vi "sim_MmW_GetAttributes.vi"(8 "error in (no error)":errorcluster, 10 "return data? (T)":bool=TRUE, 11 "reference in":refnum<class "sim_MmW.lvclass">) -> (0 "error out":errorcluster, 1 "attributes":T1={"RF config"={"TX.Frequency"=0.0, "TX.Gain"=-10.0, "TX.mmWave adapter"="mmWave1/0", "RX.Frequency"=76000000000.0, "RX.Gain"=0.0, "RX.mmWave adapter"="mmWave0/0"}, "RX samples"=0, "Downloaded Bursts"={}, "TX Fs"=0.0, "RX Fs"=0.0, "burst sequence"=[], "Burst mode"=enum."burst"} {"RF config"."RX.Frequency" format="%#_6pHz"; "RF config"."RX.Gain" format="%#_6fdb"; "RF config"."TX.Frequency" format="%#_6pHz"; "RF config"."TX.Gain" format="%#_6pHz"}, 2 "attributes ref":T4, 3 "reference out":refnum<class "sim_MmW.lvclass">)   [LabVIEW 2019, in "sim_MmW.lvclass"]
doc: "Returns a reference and if wanted the actual data values of the attributes. This method is used by the subclasses to access parent attributes."
uses:
  sim_MmW.lvclass
  C:/Program Files/National Instruments/LabVIEW 2019/vi.lib/addons/_AddQ/G#Object/G#Object.lvclass
  ObjectAttributesRef.ctl
  protected/ObjectAttributes.ctl
  mmWave HW Control/HW TXRX RF config cluster.ctl
  mmWave data_class/mmWave data.lvclass
  mmWave instrument_class/BurstMode.ctl
  sim_MmW.lvclass/sim_MmW.ctl
  <vilib>/addons/_AddQ/G#Object/G#Object.lvclass
  mmWave HW Control/mmWave HW Control.lvlib
  mmWave instrument_class/mmWave instrument.lvclass
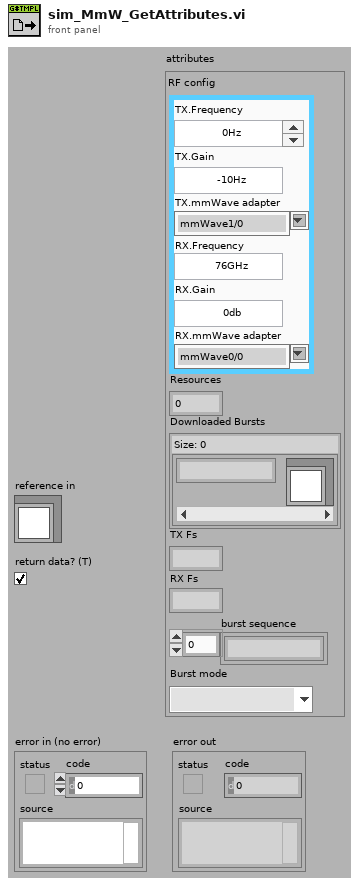
[diagram p1: front panel]
types:
  T1 = typedef "sim_MmW.lvclass/ObjectAttributes.ctl" = cluster{"RF config":T2, "RX samples":i32, "Downloaded Bursts":map{string, refnum<class "mmWave data.lvclass">}, "TX Fs":dbl, "RX Fs":dbl, "burst sequence":string[], "Burst mode":T3}
  T2 = typedef "mmWave HW Control.lvlib/HW TXRX RF config cluster.ctl" = cluster{"TX.Frequency":dbl, "TX.Gain":dbl, "TX.mmWave adapter":string, "RX.Frequency":dbl, "RX.Gain":dbl, "RX.mmWave adapter":string}
  T3 = typedef "mmWave instrument.lvclass/BurstMode.ctl" = enum16{"burst", "continuous"}
  T4 = typedef "sim_MmW.lvclass/ObjectAttributesRef.ctl" = refnum<data-value>
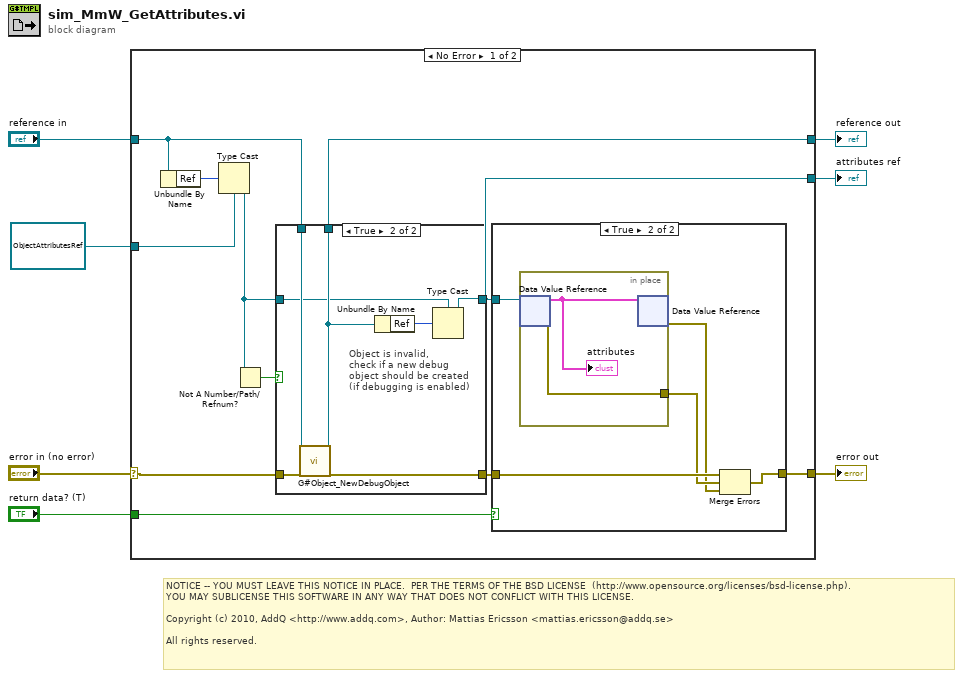
[diagram p0: block diagram]
diagram:
  # "NOTICE -- YOU MUST LEAVE THIS NOTICE IN PLACE.  PER THE TERMS OF THE BSD LICENSE  (http://www.opensource.org/licenses/bsd-license.php).\nYOU MAY SUBLICENSE THIS SOFTWARE IN ANY WAY THAT DOES NOT CONFLICT WITH THIS LICENSE.\n\nCopyright (c) 2010, AddQ <http://www.addq.com>, Author: Mattias Ericsson <mattias.ericsson@addq.se>\n\nAll rights reserved."
  n1 = case shown="No Error" "error in (no error)" {
    selector: "error in (no error)" -> [w14 w39]
    tunnel: [w17 w39] -> w6
    tunnel: [w11 w38] -> w4
    tunnel: "reference in" -> [w12 w38]
    tunnel: [w8 w37] -> w3
    tunnel: "return data? (T)" -> [w18 _]
    tunnel: T4 refnum ("attributes ref") -> [w10 w37]
    frame No Error {
      n2 = Unbundle By Name(w12) -> ("Ref"=w16:u32)
      n3 = Type Cast(type=w10, x=w16) -> (*(type *) &x=w9:T4)
      n4 = Not A Number/Path/Refnum?(number/path/refnum=w9) -> (NaN/Path/Refnum?=w13:bool)
      n5 = case shown="True" w13 {
        tunnel: [w21 w28] -> w15
        tunnel: w14 -> [w21 w27]
        tunnel: w12 -> [w20 w26]
        tunnel: [w20 w24] -> w11
        tunnel: w9 -> [w19 w23]
        tunnel: [w19 w22] -> w8
        frame False {
        }
        frame True {
          # "Object is invalid,\ncheck if a new debug\nobject should be created\n(if debugging is enabled)"
          n6 = call <vilib>:"G#Object_NewDebugObject.vi"("reference in"=w26, "error in (no error)"=w27) -> ("reference out"=w24:refnum<class "sim_MmW.lvclass">, "error out"=w28:errorcluster)  [unwired: 16 in]
          n7 = Unbundle By Name(w24) -> ("Ref"=w25:u32)
          n8 = Type Cast(type=w23, x=w25) -> (*(type *) &x=w22:T4)
        }
      }
      n9 = case shown="True" w18 {
        tunnel: w8 -> [_ w34]
        tunnel: w15 -> [w29 w33]
        tunnel: [w29 w32] -> w17
        frame False {
        }
        frame True {
          n10 = in-place {
            in-place-border: [w36] -> w31
            n11 = in-place-dvr #1(w34) -> (w35:T1, w36:errorcluster)
            "attributes" <- w35
            n12 = in-place-dvr #1(w35) -> (w30:errorcluster)  [unwired: 1 out]
          }
          n13 = Merge Errors(w33, w31, w30) -> (w32:errorcluster)
        }
      }
    }
    frame Error {
    }
  }
  "error out" <- w6
  "reference out" <- w4
  "attributes ref" <- w3
